vi "Close File.vi"(8 "error in (no error)":errorcluster, 10 "File Refnum":variant, 11 "File Manager in":refnum<class "File Abstract.lvclass">) -> (0 "error out":errorcluster, 3 "File Manager out":refnum<class "File Abstract.lvclass">)   [LabVIEW 2021, in "File Abstract.lvclass"]
doc: "This vi helps to save empty file path to class data (File Abstract.clt)"
uses:
  File Abstract.lvclass
  File Abstract.lvclass/File Abstract.ctl
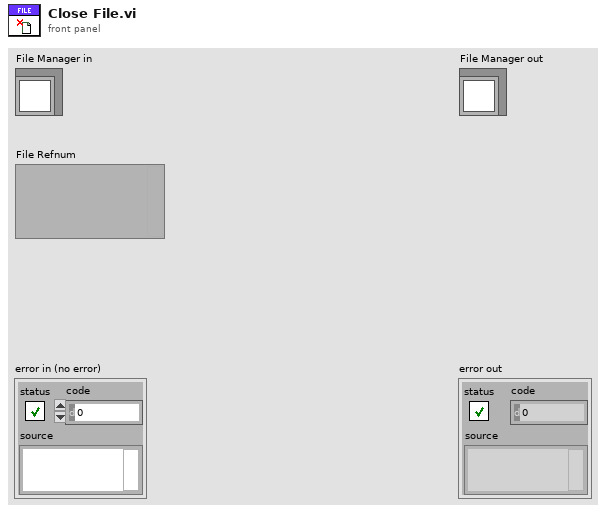
[diagram p1: front panel]
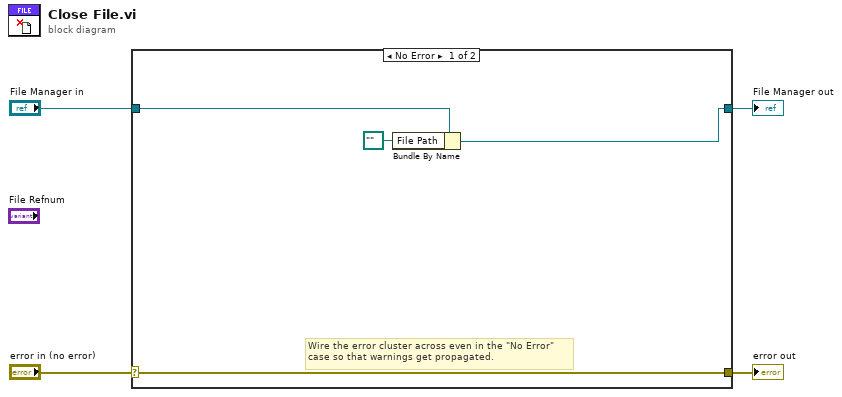
[diagram p0: block diagram]
diagram:
  n1 = case shown="No Error" "error in (no error)" {
    selector: "error in (no error)" -> [w8 w10]
    tunnel: [w8 w10] -> w3
    tunnel: [w5 w9] -> w1
    tunnel: "File Manager in" -> [w7 w9]
    frame No Error {
      # "Wire the error cluster across even in the \"No Error\"\ncase so that warnings get propagated."
      n2 = Bundle By Name(cluster=w7, "File Path"=path "") -> (w5:refnum<class "File Abstract.lvclass">)
    }
    frame Error {
    }
  }
  "error out" <- w3
  "File Manager out" <- w1
